vi "Main.vi"() -> ()   [LabVIEW 2018]
doc: "The myRIO Project template acquires acceleration data from the onboard accelerometer and displays the changes of acceleration values in a waveform chart."
uses:
  <vilib>/myRIO/Instrument Drivers/Utilities/Utilities.lvlib
  <vilib>/platform/TimedLoop/XDataNode/XDataNode.xnode
  <vilib>/Platform/TimedLoop/XDataNode/nitl_modes.ctl
  <vilib>/Platform/TimedLoop/XDataNode/XDNodeRunTimeDep.lvlib
  <vilib>/Platform/TimedLoop/XDataNode/wakeup.ctl
  <vilib>/Platform/TimedLoop/XDataNode/timing_clust.ctl
  <vilib>/myRIO/Express VI/Onboard IO/AI/AI Express VI.xnode
  <vilib>/myRIO/Instrument Drivers/Onboard IO/AI/vis/Read.vi
  <vilib>/myRIO/Instrument Drivers/Onboard IO/AI/AI.lvlib
  <vilib>/myRIO/Common/Instrument Driver Framework/Utilities/typedefs/Analog Scaling Constants.ctl
  <vilib>/myRIO/Common/Instrument Driver Framework/Utilities/typedefs/Analog Scaling Constants List.ctl
  <vilib>/myRIO/Common/Instrument Driver Framework/myRIO v1.0/AI/typedefs/AI Channels Enum.ctl
  <vilib>/myRIO/Common/Instrument Driver Framework/myRIO v1.0/AI/typedefs/AI Channels List.ctl
  <vilib>/myRIO/Common/Instrument Driver Framework/Utilities/typedefs/Generic FPGA Reference.ctl
  <vilib>/myRIO/Common/Instrument Driver Framework/Utilities/typedefs/myRIO v1.0 Reference.ctl
  <vilib>/myRIO/Common/Instrument Driver Framework/Utilities/typedefs/Hardware Version Enum.ctl
  <vilib>/myRIO/Common/Instrument Driver Framework/Utilities/typedefs/myRIO Generic Hardware Reference.ctl
  <vilib>/myRIO/Instrument Drivers/Onboard IO/AI/typedefs/AI Reference.ctl
  <vilib>/myRIO/Instrument Drivers/Onboard IO/AI/vis/myRIO AI Open.xnode
  <vilib>/myRIO/Common/Instrument Driver Framework/Utilities/vis/Is FPGA Ref Available.vi
  <vilib>/myRIO/Common/Instrument Driver Framework/myRIO v1.0/AI/vis/myRIO v1.1 Open AI.vi
  <vilib>/userdefined/High Color/nirio_resource_hc.ctl
  <vilib>/Utility/file.llb/Write Delimited Spreadsheet (DBL).vi
panel:
  in  "Frequency":dbl
  in  "input data save":path
  in  "output data save":path
  out "Thrust Forece":dbl(graph)
  out "Torque":dbl(graph)
  in  "Stop Button":bool
  out "error out":errorcluster
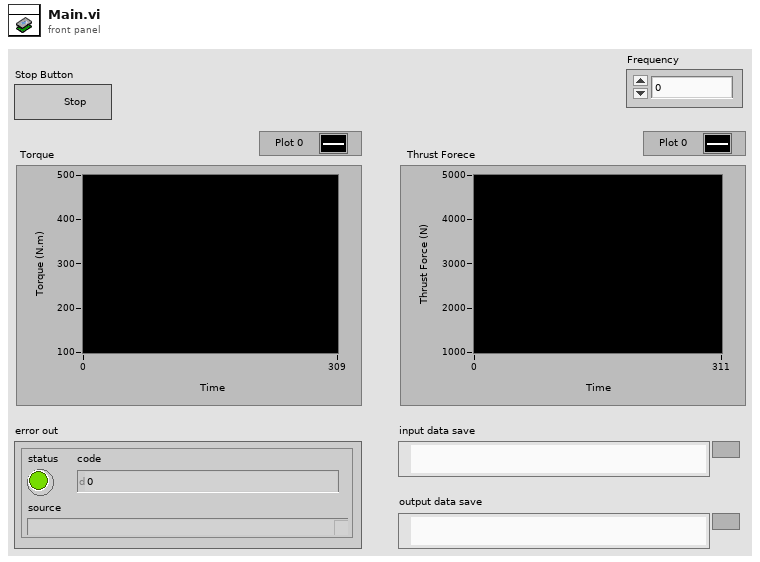
[diagram p1: front panel]
types:
  T1 = typedef "AI.lvlib/AI Reference.ctl" = cluster{"myRIO Reference":T2, "AI Channels List":T6, "AI Scaling Constants List":T8}
  T2 = typedef "myRIO Generic Hardware Reference.ctl" = cluster{"myRIO Model":T3, "myRIO Hardware Reference":T4}
  T3 = typedef "Hardware Version Enum.ctl" = enum16{"Unknown", "myRIO-1900", "myRIO-1950", "roboRIO", "NI ELVIS RIO CM", "ELVIS III"}
  T4 = typedef "myRIO v1.0 Reference.ctl" = cluster{"Generic FPGA Reference":T5, "Allow multiple opens":bool}
  T5 = typedef "Generic FPGA Reference.ctl" = refnum<k20>
  T6 = typedef "AI Channels List.ctl" = T7[]
  T7 = typedef "AI Channels Enum.ctl" = enum16{"Not Connected", "AudioIn/Left", "AudioIn/Right", "C/AI0", "C/AI1", "A/AI0", "A/AI1", "A/AI2", "A/AI3", "A/AI4", "A/AI5", "A/AI6", "A/AI7", "B/AI0", "B/AI1", "B/AI2", "B/AI3", "B/AI4", "B/AI5", "B/AI6", "B/AI7", "AI/AI0", "AI/AI1", "AI/AI2", "AI/AI3", "A/AI0 (DIFF)", "A/AI1 (DIFF)", "A/AI2 (DIFF)", "A/AI3 (DIFF)", "B/AI0 (DIFF)", "B/AI1 (DIFF)", "B/AI2 (DIFF)", "B/AI3 (DIFF)"}
  T8 = typedef "Analog Scaling Constants List.ctl" = T9[]
  T9 = typedef "Analog Scaling Constants.ctl" = cluster{"LSB Weight (Volts)":dbl, "Offset (Volts)":dbl, "Signed?":bool}
  T10 = typedef "nirio_resource_hc.ctl" = tag
  T11 = typedef "XDNodeRunTimeDep.lvlib/timing_clust.ctl" = cluster{"Expected End [f-1]":u64, "Actual End [f-1]":u64, "Finished Late? [f-1]":bool, "Expected End [i-1]":u64, "Actual End [i-1]":u64, "Finished Late? [i-1]":bool, "Expected Start [i]":u64, "Actual Start [i]":u64, "Expected Start [f]":u64, "Actual Start [f]":u64, "Source Name":string, "Structure Name":string, "Period":i64, "Deadline":i64, "Offset":i64, "Start":i64, "Priority":i32, "Timeout":i32, "Mode":T12, "Wakeup Reason":T13, "Error":errorcluster, "Source Type":string, "Secondary Source Type":string, "Global End Time":u64, "Global Start Time":u64, "Frame Duration":u64, "Iteration Duration":u64, "Assigned CPU":i32, "I/O Scan Engine Mode":u32}
  T12 = typedef "XDNodeRunTimeDep.lvlib/nitl_modes.ctl" = enum32{"No Change", "Process missed periods, maintain original phase", "Discard missed periods, maintain original phase", "Process missed periods, ignore original phase", "Discard missed periods, ignore original phase"}
  T13 = typedef "XDNodeRunTimeDep.lvlib/wakeup.ctl" = enum32{"Normal", "Aborted", "Asynchronous wakeup", "Timing source error", "Timed loop error", "Timeout"}
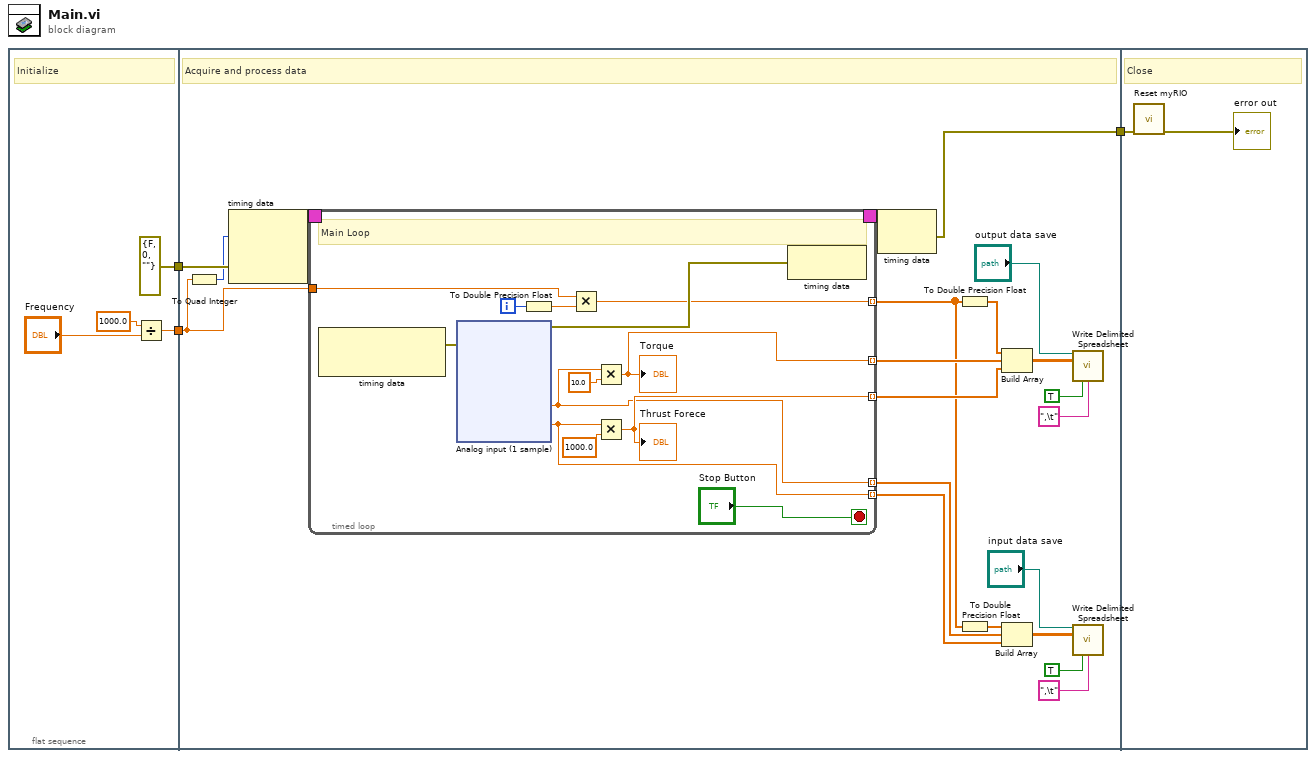
[diagram p0: block diagram]
diagram:
  n1 = flat-sequence {
    tunnel: [errorcluster {"status"=FALSE, "code"=0, "source"=""} ("error in (no error)")] -> w3
    tunnel: [w6] -> w1
    tunnel: w3 -> [w26]
    tunnel: [w16] -> w2
    tunnel: w1 -> [w25]
    tunnel: w2 -> [w91]
    frame #0 {
      # "Initialize"
      n2 = Divide(x=1000.0, y="Frequency") -> (x/y=w6:dbl)
    }
    frame #1 {
      # "Acquire and process data"
      n3 = To Quad Integer(1:w25) -> (0:w24:i64)
      n4 = node-c288(w24, w26) -> (w28:T11)  [unwired: 1 in]
      n5 = timed-loop {
        timing: w28 -> [_]
        timing-out: [_] -> w27
        tunnel: [w37] -> w22 mode=indexing
        tunnel: w25 -> [w36]
        tunnel: [w35] -> w11 mode=indexing
        tunnel: [w34] -> w21 mode=indexing
        tunnel: [w33] -> w10 mode=indexing
        tunnel: [w32] -> w9 mode=indexing
        i -> [w31]
        stop <- "Stop Button" stop-if-true
        # "Main Loop"
        n6 = node-c288() -> (w41:errorcluster)  [unwired: 1 in, 1 out]
        n7 = xnode "Analog input (1 sample)"("error in (no error)"=w41) -> ("Torque (C/AI0 (AI0))"=w33:dbl, "Thrust Forece (C/AI1 (AI1))"=w32:dbl, "error out"=w40:errorcluster)
        n8 = To Double Precision Float(number=w31) -> (double precision float=w30:dbl)
        n9 = Multiply(x=w36, y=w30) -> (x*y=w35:dbl)
        n10 = Multiply(x=w33, y=10.0 ("x")) -> (x*y=w37:dbl)
        "Torque" <- w37
        n11 = Multiply(x=w32, y=1000.0 ("x")) -> (x*y=w34:dbl)
        "Thrust Forece" <- w34
        n12 = node-c288(w40) -> ()  [unwired: 1 out]
      }
      n13 = node-c288(w27) -> (w16:errorcluster)
      n14 = To Double Precision Float(number=w11) -> (double precision float=w23:dbl[])
      n15 = To Double Precision Float(number=w11) -> (double precision float=w15:dbl[])
      n16 = Build Array(w23, w22, w21) -> (w20:dbl[][])
      n17 = Build Array(w15, w10, w9) -> (w8:dbl[][])
      n18 = call-poly <vilib>:"Write Delimited Spreadsheet.vi"("file path (dialog if empty)"="output data save", "2D data"=w20, "transpose? (no:F)"=TRUE, "delimiter (\\t)"=",\t" ("delimiter (\\t)")) -> ()  [unwired: 10 in, 2 out]
      n19 = call-poly <vilib>:"Write Delimited Spreadsheet.vi"("file path (dialog if empty)"="input data save", "2D data"=w8, "transpose? (no:F)"=TRUE, "delimiter (\\t)"=",\t" ("delimiter (\\t)")) -> ()  [unwired: 10 in, 2 out]
    }
    frame #2 {
      # "Close"
      n20 = call <vilib>:"Reset myRIO.vi"("error in (no error)"=w91) -> ("error out"=→"error out":errorcluster)  [unwired: 10 in]
    }
  }
